vi "Close.vi"(8 "error in":errorcluster, 9 "timeout (-1)":i32=-1, 11 "Standard Engine in":refnum<class "synchronous engine runtime.lvclass">) -> (0 "error out":errorcluster)   [LabVIEW 2013, in "synchronous engine runtime.lvclass"]
uses:
  synchronous engine runtime.lvclass
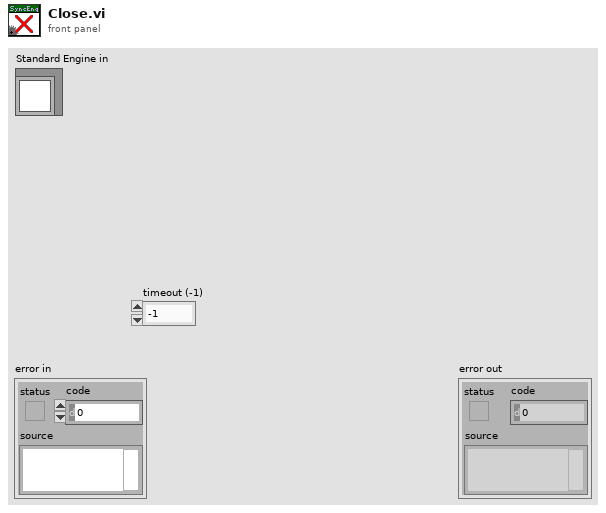
[diagram p1: front panel]
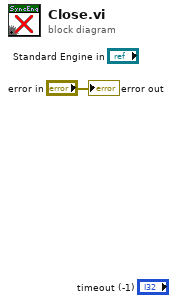
[diagram p0: block diagram]
diagram:
  "error out" <- "error in"
